vi "Tap Contour (SubVI).vi"(6 "Contour XY":u32, 8 "Complete?":bool, 10 "Input Valid?":bool) -> ()   [LabVIEW 2015]
uses:
  <vilib>/rvi/interface/RandomDataEmulation/niFpgaRandomDataHandleErrors.vi
  <vilib>/rvi/DataTransferAndStorage/Container/XNode/niFpgaContainer.xnode
  <vilib>/rvi/interface/RandomDataEmulation/nirviRandomDataFpgaReadWriteTemplate.vi
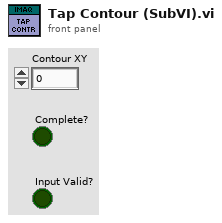
[diagram p1: front panel]
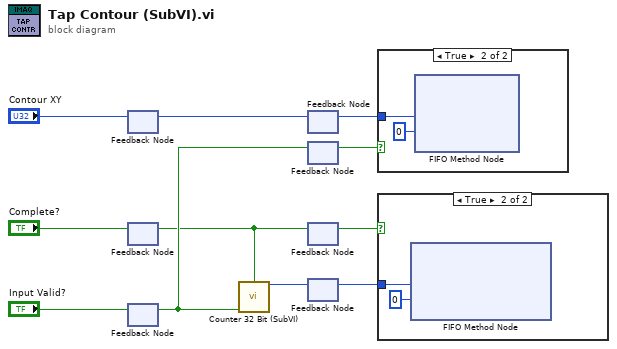
[diagram p0: block diagram]
diagram:
  n1 = feedback-in #1("Contour XY") -> ()
  n2 = feedback #1() -> (w8:u32)  [unwired: 1 in]
  n3 = feedback-in #2("Complete?") -> ()
  n4 = feedback #2() -> (w1:bool)  [unwired: 1 in]
  n5 = feedback-in #3("Input Valid?") -> ()
  n6 = feedback #3() -> (w3:bool)  [unwired: 1 in]
  n7 = call "Counter 32 Bit (SubVI).vi"("RESET"=w1, "Enable"=w3) -> ("Count"=w2:u32)  [unwired: 11 in, 2 out]
  n8 = feedback-in #4(w8) -> ()
  n9 = feedback #4() -> (w7:u32)  [unwired: 1 in]
  n10 = feedback-in #5(w3) -> ()
  n11 = feedback #5() -> (w4:bool)  [unwired: 1 in]
  n12 = feedback-in #6(w1) -> ()
  n13 = feedback #6() -> (w6:bool)  [unwired: 1 in]
  n14 = feedback-in #7(w2) -> ()
  n15 = feedback #7() -> (w5:u32)  [unwired: 1 in]
  n16 = case shown="True" w4 {
    tunnel: w7 -> [_ w13]
    frame False {
    }
    frame True {
      n17 = xnode ("FIFO Method Node")("Element"=w13, "Timeout"=0) -> ()  [unwired: 1 in, 2 out]
    }
  }
  n18 = case shown="True" w6 {
    tunnel: w5 -> [_ w15]
    frame False {
    }
    frame True {
      n19 = xnode ("FIFO Method Node")("Element"=w15, "Timeout"=0) -> ()  [unwired: 1 in, 2 out]
    }
  }
